vi "CStringToRStrings.vi"(0 "Complex string":string, 7 "Offset":i32 caption="Offset (0)", 11 "Error in":errorcluster caption="Error in (no error)") -> (4 "Real string":string, 6 "Imaginary string":string, 15 "Error out":errorcluster)   [LabVIEW 2017, in "GPString.lvlib"]
doc: "Converts <B>Complex string</B> into its <B>Real string</B> and <B>Imaginary string</B> parts, starting the conversion from the optional <B>Offset</B> in <B>Complex string</B>.\n\nSupported <B>Complex string</B> formats:\n\"(re;im)\" (radix point = \",\"), example: \"(7,8;-9)\"\n\"(re,im)\" (radix point = \".\"), example: \"(7.8,-9)\"\n\"re+im*i\" or \"re+im*j\" (radix either \".\" or \",\"), example: \"7,8-9*i\"\n\"re+imi\" or \"re+imj\" (radix either \".\" or \",\"), example: \"7.8-9j\"\n\nRe or im part only is also valid: \"re\", \"im*i\" or \"im*j\", and \"imi\" or \"imj\".\n\nThis VI is inlined.\n\nSteen Schmidt\nGPower\n15/6 2016"
uses:
  GPString.lvlib
panel:
  # "Copyright © 2016\nGPower\nSee enclosed license file for terms and conditions"
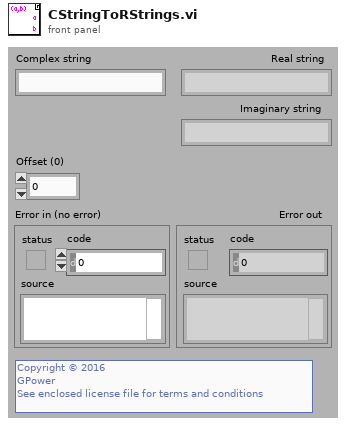
[diagram p1: front panel]
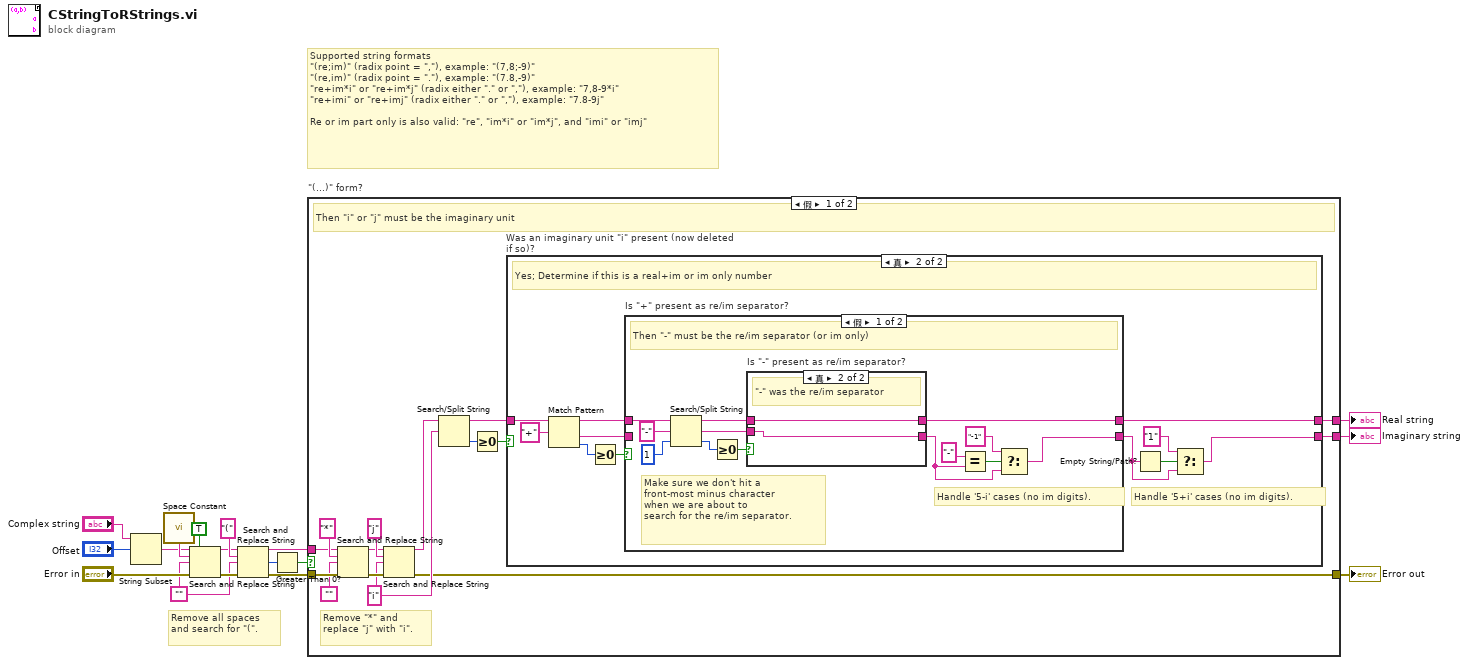
[diagram p0: block diagram]
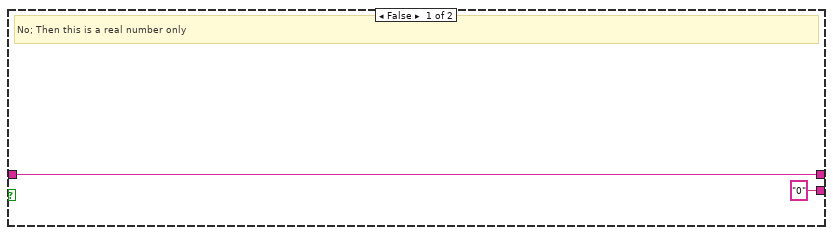
[diagram p2: hidden frame]
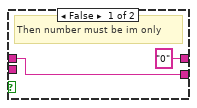
[diagram p3: hidden frame]
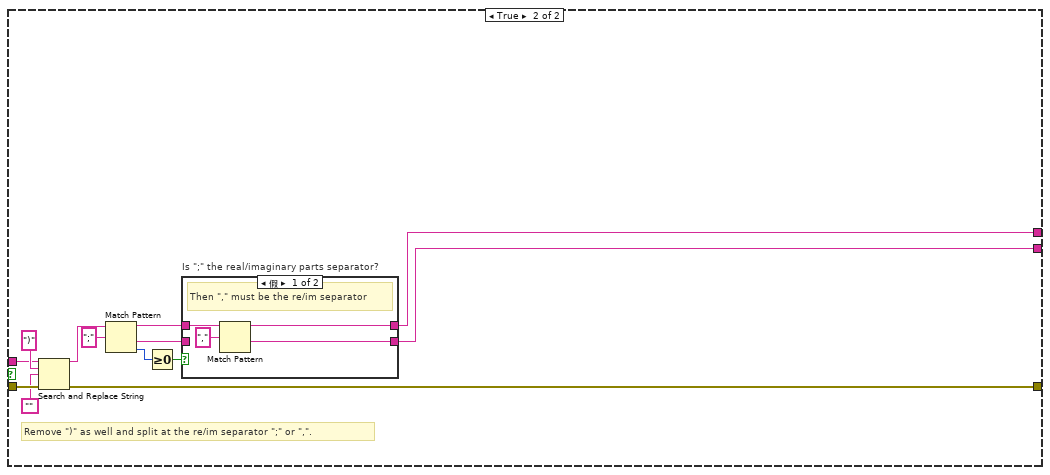
[diagram p5: hidden frame]
diagram:
  w7 = ""
  # "Remove all spaces\nand search for \"(\"."
  # "Supported string formats\n\"(re;im)\" (radix point = \",\"), example: \"(7,8;-9)\"\n\"(re,im)\" (radix point = \".\"), example: \"(7.8,-9)\"\n\"re+im*i\" or \"re+im*j\" (radix either \".\" or \",\"), example: \"7,8-9*i\"\n\"re+imi\" or \"re+imj\" (radix either \".\" or \",\"), example: \"7.8-9j\"\n\nRe or im part only is also valid: \"re\", \"im*i\" or \"im*j\", and \"imi\" or \"imj\""
  n1 = String Subset(string="Complex string", offset (0)="Offset") -> (substring=w2:string)  [unwired: 1 in]
  n2 = call <vilib>:"Space Constant.vi"() -> ("String"=w10:string)
  n3 = Search and Replace String(replace all?=TRUE ("replace all? (F)"), input string=w2, search string=w10, replace string=w7, error in="Error in") -> (result string=w5:string, error out=w8:errorcluster)  [unwired: 3 in, 2 out]
  n4 = Search and Replace String(input string=w5, search string="(", replace string=w7, error in=w8) -> (result string=w15:string, number of replacements=w14:i32, error out=w16:errorcluster)  [unwired: 4 in, 1 out]
  n5 = Greater Than 0?(x=w14) -> (x > 0?=w13:bool)
  n6 = case "\"(...)\" form?" shown="假" w13 {
    tunnel: w16 -> [w28 w76]
    tunnel: w15 -> [w27 w75]
    tunnel: [w18 w67] -> w12
    tunnel: [w19 w66] -> w11
    tunnel: [w23 w65] -> w4
    frame False {
      w25 = "i" ("search string")
      # "Remove \"*\" and\nreplace \"j\" with \"i\"."
      # "Then \"i\" or \"j\" must be the imaginary unit"
      n7 = Search and Replace String(input string=w27, search string="*", replace string="", error in=w28) -> (result string=w31:string, error out=w30:errorcluster)  [unwired: 4 in, 2 out]
      n8 = Search and Replace String(input string=w31, search string="j", replace string=w25, error in=w30) -> (result string=w24:string, error out=w23:errorcluster)  [unwired: 4 in, 2 out]
      n9 = Search/Split String(string=w24, search string/char (-)=w25) -> (substring before match=w20:string, offset of match=w22:i32)  [unwired: 1 in, 1 out]
      n10 = Greater Or Equal To 0?(x=w22) -> (x >= 0?=w21:bool)
      n11 = case "Was an imaginary unit \"i\" present (now deleted if so)?" shown="真" w21 {
        tunnel: w20 -> [w34 w40]
        tunnel: [w34 w39] -> w18
        tunnel: ["0" ("result string") w36] -> w19
        frame False {
          # "No; Then this is a real number only"
        }
        frame True {
          # "Handle '5+i' cases (no im digits)."
          # "Yes; Determine if this is a real+im or im only number"
          n12 = Match Pattern(string=w40, regular expression="+") -> (before substring=w42:string, after substring=w41:string, offset past match=w44:i32)  [unwired: 1 in, 1 out]
          n13 = Greater Or Equal To 0?(x=w44) -> (x >= 0?=w43:bool)
          n14 = case "Is \"+\" present as re/im separator?" shown="假" w43 {
            tunnel: w42 -> [w55 w64]
            tunnel: w41 -> [_ w63]
            tunnel: [w51 w64] -> w39
            tunnel: [w47 w63] -> w35
            frame False {
              # "Handle '5-i' cases (no im digits)."
              # "Make sure we don't hit a\nfront-most minus character\nwhen we are about to\nsearch for the re/im separator."
              # "Then \"-\" must be the re/im separator (or im only)"
              n15 = Search/Split String(string=w55, search string/char (-)="-" ("regular expression"), offset (0)=1) -> (substring before match=w52:string, match + rest of string=w53:string, offset of match=w54:i32)
              n16 = Greater Or Equal To 0?(x=w54) -> (x >= 0?=w58:bool)
              n17 = case "Is \"-\" present as re/im separator?" shown="真" w58 {
                tunnel: w52 -> [w60 w62]
                tunnel: w53 -> [_ w61]
                tunnel: ["0" ("result string") w62] -> w51
                tunnel: [w60 w61] -> w46
                frame False {
                  # "Then number must be im only"
                }
                frame True {
                  # "\"-\" was the re/im separator"
                }
              }
              n18 = Equal?(x="-", y=w46) -> (x = y?=w50:bool)
              n19 = Select(t="-1", s=w50, f=w46) -> (s? t:f=w47:string)
            }
            frame True {
              # "\"+\" was the re/im separator"
            }
          }
          n20 = Empty String/Path?(string/path=w35) -> (empty?=w37:bool)
          n21 = Select(t="1", s=w37, f=w35) -> (s? t:f=w36:string)
        }
      }
    }
    frame True {
      # "Remove \")\" as well and split at the re/im separator \";\" or \",\"."
      n22 = Search and Replace String(input string=w75, search string=")", replace string="", error in=w76) -> (result string=w73:string, error out=w65:errorcluster)  [unwired: 4 in, 2 out]
      n23 = Match Pattern(string=w73, regular expression=";") -> (before substring=w69:string, after substring=w68:string, offset past match=w71:i32)  [unwired: 1 in, 1 out]
      n24 = Greater Or Equal To 0?(x=w71) -> (x >= 0?=w70:bool)
      n25 = case "Is \";\" the real/imaginary parts separator?" shown="假" w70 {
        tunnel: w69 -> [w80 w83]
        tunnel: w68 -> [_ w82]
        tunnel: [w79 w83] -> w67
        tunnel: [w78 w82] -> w66
        frame False {
          # "Then \",\" must be the re/im separator"
          n26 = Match Pattern(string=w80, regular expression=",") -> (before substring=w79:string, after substring=w78:string)  [unwired: 1 in, 2 out]
        }
        frame True {
          # "\";\" was the re/im separator"
        }
      }
    }
  }
  "Error out" <- w4
  "Real string" <- w12
  "Imaginary string" <- w11
